vi "Msg_to_LEDs.vi"(0 "SingleBoard?":bool, 7 "ERD Data Out":cluster{"ERD Number":u16, "Data":string}[](array[cluster]) {"ERD Number" format="%.0x"}) -> (4 "Convert raw data":string[](array[string]), 6 "Justice League UI":T1, 8 "Justice League SB":T2, 10 "LED's Out 0-79":bool[](array[boolean]))   [LabVIEW 2016]
uses:
  type defs/UI_LEDs.ctl
  type defs/SB_LEDs.ctl
panel:
  out "Error Out":errorcluster
  in  "Error In":errorcluster
  in  "Tab Control":enum32{"UI/MC", "SingleBoard"}(tab)
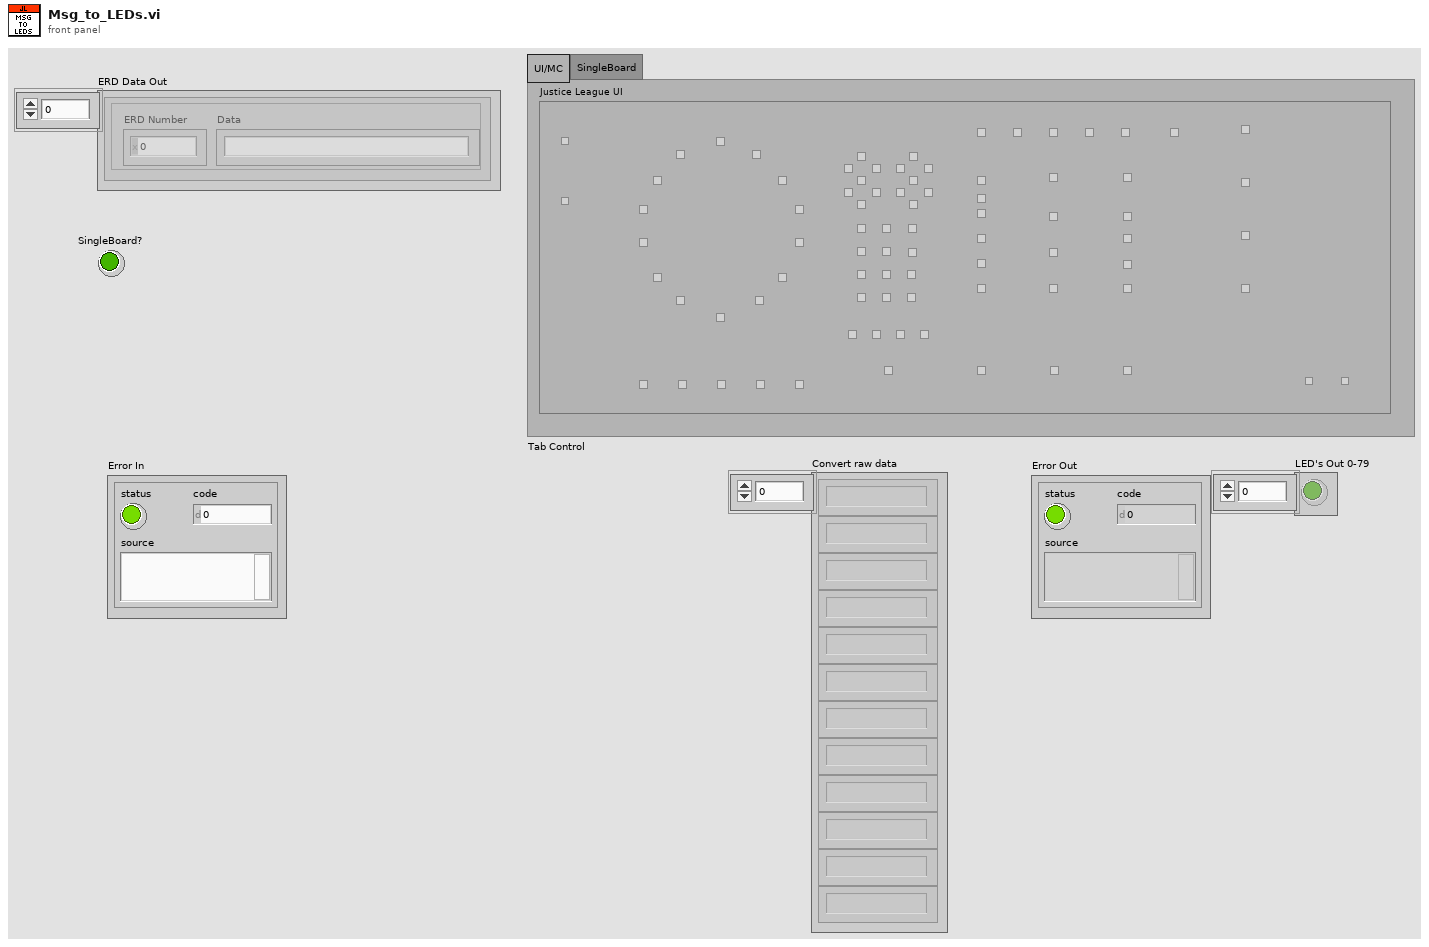
[diagram p1: front panel]
types:
  T1 = typedef "UI_LEDs.ctl" = cluster{"Z301 - Encoder 0":bool, "Z302 - Encoder 13":bool, "Z303 - Encoder 12":bool, "Z304 - Encoder 11":bool, "Z305 - Encoder 10":bool, "Z306 - Encoder 09":bool, "Z307 - Encoder 08":bool, "Z308 - Encoder 07":bool, "Z309 - Encoder 06":bool, "Z310 - Encoder 05":bool, "Z311 - Encoder 04":bool, "Z312 - Encoder 03":bool, "Z313 - Encoder 02":bool, "Z314 - Encoder 01":bool, "Z315 - Unpopulated":bool, "Z316 - Unpopulated":bool, "Z317 - SSD1:A":bool, "Z318 - SSD1:B":bool, "Z319 - SSD1:G":bool, "Z320 - SSD1:C":bool, "Z321 - SSD1:D":bool, "Z322 - SSD1:E":bool, "Z323 - SSD1:F":bool, "Z324 - Pause 1":bool, "Z325 - Control Lock 1":bool, "Z326 - Sensing 1":bool, "Z327 - Clean Lint Filter 1":bool, "Z328 - Extra Status 1":bool, "Z329 - Extra Status 2":bool, "Z330 - Clean Lint Filter 2":bool, "Z331 -Sensing 2":bool, "Z332 - Unpopulated":bool, "Z333 - SSD2:A":bool, "Z334 - SSD2:B":bool, "Z335 - SSD2:G":bool, "Z345 - SSD2:C":bool, "Z336 - SSD2:D":bool, "Z337 - SSD2:E":bool, "Z338 - SSD2:F":bool, "Z339 - Pause 3":bool, "Z340 - Control Lock 3":bool, "Z353 - Sensing 3":bool, "Z342 - Clean Lint Filter 3":bool, "Z344 - Extra Status 3":bool, "Z346 - Extra Status 4":bool, "Z341 - Pause 2":bool, "Z343 - Control Lock 2":bool, "Z347 - Unpopulated":bool, "Z348 -My Cycle":bool, "Z349 - Delay Dry":bool, "Z350 - Volume":bool, "Z351 - Damp Alert":bool, "Z352 - Bar 1":bool, "Z354 - Bar 2":bool, "Z355 - Bar 3":bool, "Z356 - Bar 4":bool, "Z357 - Bar 5":bool, "Z358 - eDry":bool, "Z359 - Time Increment":bool, "Z360 - Time Decrement":bool, "Z361 - Extended Tumble":bool, "Z362 - Unpopulated":bool, "Z363 - Unpopulated":bool, "Z364 - Unpopulated":bool, "Z365 - Status 1":bool, "Z366 - Status 3":bool, "Z367 - Default Time 5":bool, "Z368 - Default Time 4":bool, "Z369 - Default Time 3":bool, "Z370 - Dry":bool, "Z371 - Status 2":bool, "Z372 -Default Time 2":bool, "Z373 - Default Time 1":bool, "Z374 - Unpopulated":bool, "Z375 - Default Time 0":bool, "Z376 - No Heat":bool, "Z377 - Unpopulated":bool, "Z378 - Unpopulated":bool, "Z379 - Unpopulated":bool, "Z380 - Unpopulated":bool, "Z381 - Status 4":bool, "Z382 - Status 6":bool, "Z383 - More Dry":bool, "Z384 - High":bool, "Z385 - Medium":bool, "Z386 -Low":bool, "Z387 - Status 5":bool, "Z388 - Less Dry":bool, "Z388 - Extra Low":bool, "Z390 - Unpopulated":bool, "Z391 - Damp":bool, "Z392 - Unpopulated":bool, "Z393 - Unpopulated":bool, "Z394 - Unpopulated":bool, "Z395 - Unpopulated":bool, "Z396 - Unpopulated":bool, "Z101 - unpop?":bool, "Z102 - Start/Pause":bool, "OFF - OFF":bool, "MAX - MAX":bool}
  T2 = typedef "SB_LEDs.ctl" = cluster{"Z101 - Start/Pause":bool, "Z - unpop?":bool, "Z103 - Encoder 0":bool, "Z104 - Encoder 13":bool, "Z105 - Encoder 12":bool, "Z106 - Encoder 11":bool, "Z107 - Encoder 10":bool, "Z108 - Encoder 09":bool, "Z109 - Encoder 08":bool, "Z110 - Encoder 07":bool, "Z111 - Encoder 06":bool, "Z112 - Encoder 05":bool, "Z113 - Encoder 04":bool, "Z114 - Encoder 03":bool, "Z115 - Encoder 02":bool, "Z116 - Encoder 01":bool, "Z117 - Bar 1":bool, "Z118 - Bar 2":bool, "Z119 - Bar 3":bool, "Z120 - Bar 4":bool, "Z121 - Bar 5":bool, "Z122 - SSD1:A":bool, "Z123 - SSD1:B":bool, "Z124 - SSD1:C":bool, "Z125 - SSD1:D":bool, "Z126 - SSD1:E":bool, "Z127 - SSD1:F":bool, "Z128 - SSD1:G":bool, "Z129 - SSD2:A":bool, "Z130 - SSD2:B":bool, "Z131 - SSD2:C":bool, "Z132 - SSD2:D":bool, "Z133 - SSD2:E":bool, "Z134 - SSD2:F":bool, "Z135 - SSD2:G":bool, "Z136 - Pause 2":bool, "Z137 - Pause 3":bool, "Z138 - Control Lock 1":bool, "Z139 - Control Lock 2":bool, "Z140 - Control Lock 3":bool, "Z142 - Sensing 1":bool, "Z142 -Sensing 2":bool, "Z143 - Sensing 3":bool, "Z144 - Extra Status 1":bool, "Z145 - Extra Status 2":bool, "Z146 - Extra Status 3":bool, "Z147 - Extra Status 4":bool, "Z148 - Status 1":bool, "Z149 - Status 2":bool, "Z150 - Status 3":bool, "Z151 - Status 4":bool, "Z152 - Status 5":bool, "Z153 - Status 6":bool, "Z154 - Default Time 5":bool, "Z155 - Default Time 4":bool, "Z153 - Default Time 3":bool, "Z157 -Default Time 2":bool, "Z158 - Default Time 1":bool, "Z159 - Default Time 0":bool, "Z160 - More Dry":bool, "Z161 - Dry":bool, "Z162 - Less Dry":bool, "Z163 - Damp":bool, "Z164 - High":bool, "Z165 - Medium":bool, "Z166 - Extra Low":bool, "Z167 - No Heat":bool, "Z168 - Volume":bool, "Z169 - Damp Alert":bool, "Z170 - Extended Tumble":bool, "Z171 - Time Decrement":bool, "Z172 - Time Increment":bool, "Z173 - eDry":bool, "Z174 -My Cycle":bool, "Z175 - Delay Dry":bool, "Z176 - Clean Lint Filter 1":bool, "Z177 - Clean Lint Filter 2":bool, "Z178 - Clean Lint Filter 3":bool, "Z179 - Pause 1":bool, "OFF - OFF":bool, "MAX - MAX":bool, "Z165B -Low":bool}
  T3 = cluster{"[0]":bool, "[1]":bool, "[2]":bool, "[3]":bool, "[4]":bool, "[5]":bool, "[6]":bool, "[7]":bool, "[8]":bool, "[9]":bool, "[10]":bool, "[11]":bool, "[12]":bool, "[13]":bool, "[14]":bool, "[15]":bool, "[16]":bool, "[17]":bool, "[18]":bool, "[19]":bool, "[20]":bool, "[21]":bool, "[22]":bool, "[23]":bool, "[24]":bool, "[25]":bool, "[26]":bool, "[27]":bool, "[28]":bool, "[29]":bool, "[30]":bool, "[31]":bool, "[32]":bool, "[33]":bool, "[34]":bool, "[35]":bool, "[36]":bool, "[37]":bool, "[38]":bool, "[39]":bool, "[40]":bool, "[41]":bool, "[42]":bool, "[43]":bool, "[44]":bool, "[45]":bool, "[46]":bool, "[47]":bool, "[48]":bool, "[49]":bool, "[50]":bool, "[51]":bool, "[52]":bool, "[53]":bool, "[54]":bool, "[55]":bool, "[56]":bool, "[57]":bool, "[58]":bool, "[59]":bool, "[60]":bool, "[61]":bool, "[62]":bool, "[63]":bool, "[64]":bool, "[65]":bool, "[66]":bool, "[67]":bool, "[68]":bool, "[69]":bool, "[70]":bool, "[71]":bool, "[72]":bool, "[73]":bool, "[74]":bool, "[75]":bool, "[76]":bool, "[77]":bool, "[78]":bool, "[79]":bool, "[80]":bool, "[81]":bool}
  T4 = cluster{"[0]":bool, "[1]":bool, "[2]":bool, "[3]":bool, "[4]":bool, "[5]":bool, "[6]":bool, "[7]":bool, "[8]":bool, "[9]":bool, "[10]":bool, "[11]":bool, "[12]":bool, "[13]":bool, "[14]":bool, "[15]":bool, "[16]":bool, "[17]":bool, "[18]":bool, "[19]":bool, "[20]":bool, "[21]":bool, "[22]":bool, "[23]":bool, "[24]":bool, "[25]":bool, "[26]":bool, "[27]":bool, "[28]":bool, "[29]":bool, "[30]":bool, "[31]":bool, "[32]":bool, "[33]":bool, "[34]":bool, "[35]":bool, "[36]":bool, "[37]":bool, "[38]":bool, "[39]":bool, "[40]":bool, "[41]":bool, "[42]":bool, "[43]":bool, "[44]":bool, "[45]":bool, "[46]":bool, "[47]":bool, "[48]":bool, "[49]":bool, "[50]":bool, "[51]":bool, "[52]":bool, "[53]":bool, "[54]":bool, "[55]":bool, "[56]":bool, "[57]":bool, "[58]":bool, "[59]":bool, "[60]":bool, "[61]":bool, "[62]":bool, "[63]":bool, "[64]":bool, "[65]":bool, "[66]":bool, "[67]":bool, "[68]":bool, "[69]":bool, "[70]":bool, "[71]":bool, "[72]":bool, "[73]":bool, "[74]":bool, "[75]":bool, "[76]":bool, "[77]":bool, "[78]":bool, "[79]":bool, "[80]":bool, "[81]":bool, "[82]":bool, "[83]":bool, "[84]":bool, "[85]":bool, "[86]":bool, "[87]":bool, "[88]":bool, "[89]":bool, "[90]":bool, "[91]":bool, "[92]":bool, "[93]":bool, "[94]":bool, "[95]":bool, "[96]":bool, "[97]":bool, "[98]":bool, "[99]":bool}
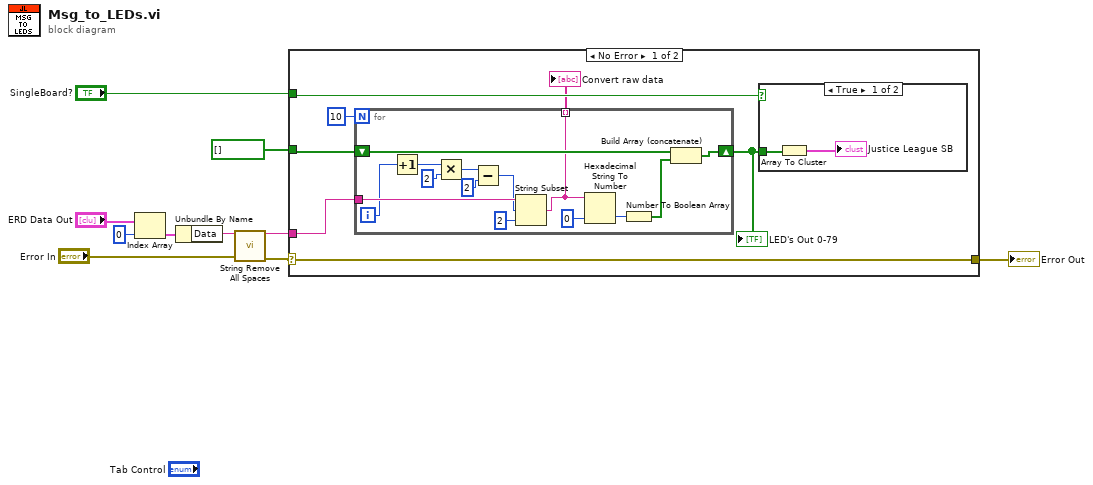
[diagram p0: block diagram]
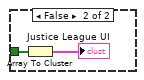
[diagram p2: hidden frame]
diagram:
  n1 = Index Array(array="ERD Data Out", index=0) -> (element=w8:cluster{"ERD Number":u16, "Data":string})
  n2 = Unbundle By Name(w8) -> ("Data"=w5:string)
  n3 = call "String Remove All Spaces.vi"("Input String"=w5, "error in (no error)"="Error In") -> ("Spaces Removed"=w6:string, "error out"=w2:errorcluster)  [unwired: 12 in]
  n4 = case shown="No Error" w2 {
    selector: w2 -> [w12 w36]
    tunnel: bool[] [] -> [w17 _]
    tunnel: w6 -> [w16 _]
    tunnel: "SingleBoard?" -> [w13 _]
    tunnel: [w12 w36] -> w1
    frame No Error {
      n5 = for {
        N: 10 -> [_]
        shift-right: [w33] -> w14
        shift-left: w17 -> [w34]
        tunnel: w16 -> [w31]
        tunnel: [w22] -> w11 mode=indexing
        i -> [w25]
        n6 = Increment(x=w25) -> (x+1=w26:i32)
        n7 = Multiply(x=w26, y=2) -> (x*y=w28:i32)
        n8 = Subtract(x=w28, y=2) -> (x-y=w24:i32)
        n9 = String Subset(string=w31, offset (0)=w24, length (rest)=2 ("length (rest)")) -> (substring=w22:string)
        n10 = Hexadecimal String To Number(string=w22, default (0uL)=u8 0) -> (number=w35:u8)  [unwired: 1 in, 1 out]
        n11 = Number To Boolean Array(number=w35) -> (Boolean array=w23:bool[])
        n12 = Build Array (concatenate)(w34, w23) -> (w33:bool[])
      }
      "Convert raw data" <- w11
      "LED's Out 0-79" <- w14
      n13 = case shown="True" w13 {
        tunnel: w14 -> [w19 w21]
        frame True {
          n14 = Array To Cluster(array=w19) -> (cluster=→"Justice League SB":T3)
        }
        frame False {
          n15 = Array To Cluster(array=w21) -> (cluster=→"Justice League UI":T4)
        }
      }
    }
    frame Error {
    }
  }
  "Error Out" <- w1
